vi "Crosstalk.vi"(6 "expected fundamental frequency [Hz]":dbl=-1.0 format="%.2f", 8 "error in (no error)":errorcluster, 10 "idle channel response":waveform(dbl)[](array[waveform]), 11 "stimulus signal":waveform(dbl)) -> (0 "error out":errorcluster, 1 "complex spectrum idle-channel response":T7(array[cluster]) {"spectrum info"."x-axis units" items=["Time (s)"=0, "Frequency-CB (Hz)"=1, "Frequency-CPB (Hz)"=1248, "Frequency-Arbitrary (Hz)"=2357, "Quefrency (s)"=2, "Revolutions (rev)"=3, "Order"=4, "Speed (RPM)"=11, "Speed (rad/s)"=21, "Index"=65535]; "spectrum info"."weighting filter" items=["Linear", "A-weighting", "B-weighting", "C-weighting", "ITU-R 468-4", "Dolby", "CCITT", "C-message", "Wb", "Wc", "Wd", "We", "Wf", "Wh", "Wj", "Wk", "Wm", "AES17 20 kHz lowpass", "AES17 40 kHz lowpass", "AES17 20 kHz highpass", "AES17 40 kHz highpass"]; "spectrum info"."dB reference [EU]" format="%.2f"; "spectrum info"."engineering units" items=["custom..."=0, "V"=1, "A"=21, "C"=30, "pC"=31, "s"=32, "-"=29, "Pa"=2, "N"=20, "g"=3, "m/s^2"=4, "m/s"=5, "m"=6, "mm/s"=12, "mm"=13, "micron/s"=14, "micron"=15, "in/s^2"=7, "in/s"=8, "in"=9, "mil/s"=10, "mil"=11, "rad/s^2"=16, "rad/s"=17, "rad"=18, "deg/s^2"=26, "deg/s"=27, "deg"=28, "RPM"=22, "cycle/s^2"=23, "Hz"=24, "cycle"=25, "strain"=19]; "spectrum info"."spectral info"."window" items=["None "=0, "Hanning"=1, "Hamming"=2, "Blackman-Harris"=3, "Exact Blackman"=4, "Blackman"=5, "Flat Top"=6, "4 Term B-Harris "=7, "7 Term B-Harris"=8, "Low Sidelobe"=9, "Force - Exponential"=10, "Gaussian"=62]}, 2 "crosstalk":dbl[](array[numeric]), 3 "complex spectrum\nstimulus X":T8={"complex spectrum response"={"f0"=0.0, "df"=1.0, "complex spectrum"=[]}, "spectrum info"={"channel name"="", "description"="", "x-axis units"=0, "spectral info"={"spectrum type"=enum."Power [Magnitude^2]", "linear/dB"=enum."linear", "window"=0, "window size"=0, "FFT size"=0}, "engineering units"=0, "custom label"="", "dB reference [EU]"=0.0, "peak units"=enum."rms", "weighting filter"=0, "spectral density?"=FALSE, "unit label"="", "spectrum skewed?"=FALSE, "complimentary spectrum units"=enum."none"}} {"spectrum info"."x-axis units" items=["Time (s)"=0, "Frequency-CB (Hz)"=1, "Frequency-CPB (Hz)"=1248, "Frequency-Arbitrary (Hz)"=2357, "Quefrency (s)"=2, "Revolutions (rev)"=3, "Order"=4, "Speed (RPM)"=11, "Speed (rad/s)"=21, "Index"=65535]; "spectrum info"."weighting filter" items=["Linear", "A-weighting", "B-weighting", "C-weighting", "ITU-R 468-4", "Dolby", "CCITT", "C-message", "Wb", "Wc", "Wd", "We", "Wf", "Wh", "Wj", "Wk", "Wm", "AES17 20 kHz lowpass", "AES17 40 kHz lowpass", "AES17 20 kHz highpass", "AES17 40 kHz highpass"]; "spectrum info"."dB reference [EU]" format="%.2f"; "spectrum info"."engineering units" items=["custom..."=0, "V"=1, "A"=21, "C"=30, "pC"=31, "s"=32, "-"=29, "Pa"=2, "N"=20, "g"=3, "m/s^2"=4, "m/s"=5, "m"=6, "mm/s"=12, "mm"=13, "micron/s"=14, "micron"=15, "in/s^2"=7, "in/s"=8, "in"=9, "mil/s"=10, "mil"=11, "rad/s^2"=16, "rad/s"=17, "rad"=18, "deg/s^2"=26, "deg/s"=27, "deg"=28, "RPM"=22, "cycle/s^2"=23, "Hz"=24, "cycle"=25, "strain"=19]; "spectrum info"."spectral info"."window" items=["None "=0, "Hanning"=1, "Hamming"=2, "Blackman-Harris"=3, "Exact Blackman"=4, "Blackman"=5, "Flat Top"=6, "4 Term B-Harris "=7, "7 Term B-Harris"=8, "Low Sidelobe"=9, "Force - Exponential"=10, "Gaussian"=62]; "complex spectrum response"."complex spectrum" format="%.2f"; "complex spectrum response"."df" format="%.2f"; "complex spectrum response"."f0" format="%.2f"}, 4 "detected tone stimulus":cluster{"frequency [Hz]":dbl, "amplitude":dbl})   [LabVIEW 2021, in "Crosstalk_Audio DAC.lvlib"]
uses:
  Crosstalk_Audio DAC.lvlib
  <vilib>/addons/_NISVFA/_Shared subVIs/Controls/svc_Spectrum Info.ctl
  <vilib>/addons/_NISVFA/_Shared subVIs/Controls/svc_X-Axis Units.ctl
  <vilib>/addons/_NISVFA/_Shared subVIs/Controls/svc_Spectrum Type.ctl
  <vilib>/addons/_NISVFA/_Shared subVIs/Controls/svc_Engineering Units Text Ring.ctl
  <vilib>/addons/_NISVFA/_Shared subVIs/Controls/svc_Weighting Filter Text Ring.ctl
  <vilib>/addons/_NISVFA/_Shared subVIs/Controls/svc_Complimentary Spectrum Units.ctl
  <vilib>/addons/_NISVFA/_Shared subVIs/Controls/svc_Window.ctl
  <vilib>/addons/Sound and Vibration/svt_Distortion/SoundVib_Distortion.lvlib
  <vilib>/addons/Sound and Vibration/svt_Single Tone Measurements/SoundVib_SingleTone.lvlib
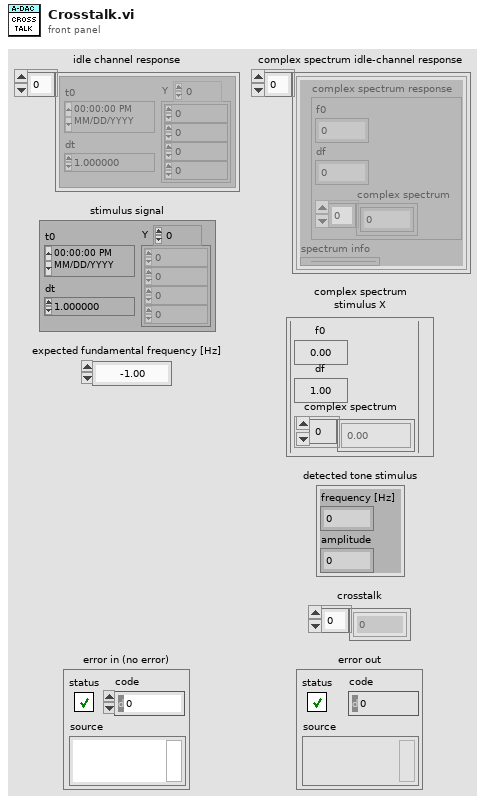
[diagram p1: front panel]
types:
  T1 = typedef "svc_Spectrum Info.ctl" = cluster{"channel name":string, "description":string, "x-axis units":T2, "spectral info":cluster{"spectrum type":T3, "linear/dB":enum16{"linear", "dB"}, "window":u16, "window size":i32, "FFT size":i32}, "engineering units":T4, "custom label":string, "dB reference [EU]":dbl, "peak units":enum16{"rms", "peak", "peak-peak"}, "weighting filter":T5, "spectral density?":bool, "unit label":string, "spectrum skewed?":bool, "complimentary spectrum units":T6}
  T2 = typedef "svc_X-Axis Units.ctl" = u16
  T3 = typedef "svc_Spectrum Type.ctl" = enum16{"FFT Spectrum [complex]", "Amplitude [Magnitude]", "Power [Magnitude^2]", "Cross Spectrum [complex]", "Frequency Response [Complex]"}
  T4 = typedef "svc_Engineering Units Text Ring.ctl" = u16
  T5 = typedef "svc_Weighting Filter Text Ring.ctl" = u16
  T6 = typedef "svc_Complimentary Spectrum Units.ctl" = enum16{"none", "radians", "degrees", "cycles", "imaginary"}
  T7 = cluster{"complex spectrum response":cluster{"f0":dbl, "df":dbl, "complex spectrum":cdb[]}, "spectrum info":T1}[]
  T8 = cluster{"complex spectrum response":cluster{"f0":dbl, "df":dbl, "complex spectrum":cdb[]}, "spectrum info":T1}
  T9 = typedef "svc_Window.ctl" = u32
  T10 = cluster{"complex spectrum":cluster{"f0":dbl, "df":dbl, "complex spectrum":cdb[]}, "spectrum info":T1}
  T11 = cluster{"complex spectrum":cluster{"f0":dbl, "df":dbl, "complex spectrum":cdb[]}, "spectrum info":T1}[]
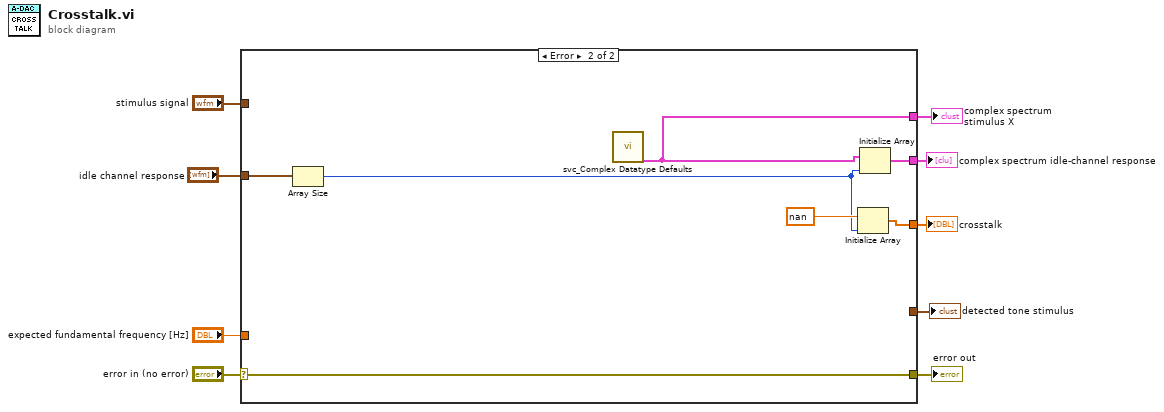
[diagram p0: block diagram]
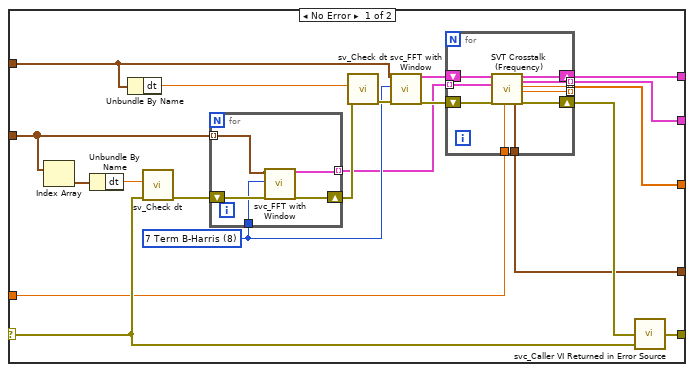
[diagram p2: hidden frame]
diagram:
  n1 = case shown="Error" "error in (no error)" {
    selector: "error in (no error)" -> [w15 w51]
    tunnel: "idle channel response" -> [w12 w50]
    tunnel: "stimulus signal" -> [w16 _]
    tunnel: [w26 w51] -> w8
    tunnel: [w28 w46] -> w2
    tunnel: [w23 w48] -> w3
    tunnel: [w24 w49] -> w6
    tunnel: "expected fundamental frequency [Hz]" -> [w14 _]
    tunnel: [w10 _] -> w1
    frame No Error {
      w19 = T9 8 items=["None ", "Hanning", "Hamming", "Blackman-Harris", "Exact Blackman", "Blackman", "Flat Top", "4 Term B-Harris ", "7 Term B-Harris", "Low Sidelobe"] ("window")
      n2 = Index Array(array=w12) -> (element=w13:waveform(dbl))  [unwired: 1 in]
      n3 = Unbundle By Name(w13) -> ("dt"=w17:dbl)
      n4 = Unbundle By Name(w16) -> ("dt"=w18:dbl)
      n5 = call <vilib>:"sv_Check dt.vi"("error in"=w15, "dt"=w17) -> ("error out"=w22:errorcluster)  [unwired: 8 in, 1 out]
      n6 = for {
        tunnel: w19 -> [w42]
        shift-right: [w43] -> w21
        shift-left: w22 -> [w44]
        tunnel: w12 -> [w41] mode=indexing
        tunnel: [w40] -> w11 mode=indexing
        n7 = call <vilib>:"svc_FFT with Window.vi"("time signal in [EU]"=w41, "window"=w42, "error in"=w44) -> ("complex spectrum"=w40:T8, "error out"=w43:errorcluster)  [unwired: 15 in]
      }
      n8 = call <vilib>:"sv_Check dt.vi"("error in"=w21, "dt"=w18) -> ("error out"=w20:errorcluster)  [unwired: 8 in, 1 out]
      n9 = call <vilib>:"svc_FFT with Window.vi"("time signal in [EU]"=w16, "window"=w19, "error in"=w20) -> ("complex spectrum"=w27:T8, "error out"=w25:errorcluster)  [unwired: 15 in]
      n10 = for {
        tunnel: [w38] -> w28 mode=indexing
        tunnel: [w36] -> _ mode=indexing
        tunnel: [w33] -> w23 mode=indexing
        tunnel: w14 -> [w32]
        shift-right: [w34] -> w24
        shift-left: w27 -> [w37]
        shift-right: [w39] -> w29
        shift-left: w25 -> [w35]
        tunnel: w11 -> [w31] mode=indexing
        tunnel: [w30] -> w10
        n11 = call <vilib>:"SVT Crosstalk (Frequency).vi"("complex spectrum\nstimulus X"=w37, "complex spectrum\nidle-channel response Y"=w31, "error in (no error)"=w35, "expected fundamental frequency [Hz]"=w32) -> ("detected tone stimulus"=w30:cluster{"frequency [Hz]":dbl, "amplitude":dbl}, "dup complex spectrum\nstimulus X"=w34:T8, "dup complex spectrum\nidle-channel response Y"=w33:T8, "crosstalk"=w38:dbl, "phase lag"=w36:dbl, "error out"=w39:errorcluster)  [unwired: 8 in, 2 out]
      }
      n12 = call <vilib>:"svc_Caller VI Returned in Error Source.vi"("warning input to caller"=w15, "error in"=w29) -> ("error out"=w26:errorcluster)  [unwired: 3 in]
    }
    frame Error {
      n13 = Array Size(array=w50) -> (size(s)=w45:i32)
      n14 = call <vilib>:"svc_Complex Datatype Defaults.vi"() -> ("complex spectrum"=w49:T10)  [unwired: 11 in, 8 out]
      n15 = Initialize Array(nan ("phase lag"), w45) -> (w46:dbl[])
      n16 = Initialize Array(w49, w45) -> (w48:T11)
    }
  }
  "error out" <- w8
  "complex spectrum\nstimulus X" <- w6
  "complex spectrum idle-channel response" <- w3
  "crosstalk" <- w2
  "detected tone stimulus" <- w1
